vi "Math-RMS From Magnitude Spectrum.vi"(1 "Magnitude (dB)":dbl[](array[numeric])) -> (0 "RMS (dB)":dbl)   [LabVIEW 2015]
uses:
  dB to Linear (1D).vi
  Linear to dB (scalar).vi
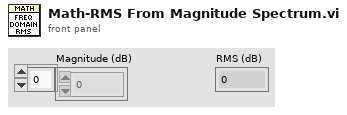
[diagram p1: front panel]
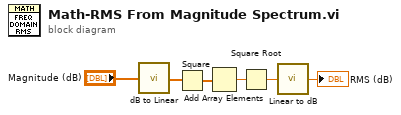
[diagram p0: block diagram]
diagram:
  n1 = call-poly "dB to Linear.vi"("dB"="Magnitude (dB)") -> ("linear"=w3:dbl[])
  n2 = Square(x=w3) -> (x^2=w4:dbl[])
  n3 = Add Array Elements(numeric array=w4) -> (sum=w5:dbl)
  n4 = Square Root(x=w5) -> (sqrt(x)=w6:dbl)
  n5 = call-poly "Linear to dB.vi"("Linear"=w6) -> ("dB"=→"RMS (dB)":dbl)
